vi "VISA init.vi"(8 "error in (no error)":errorcluster, 11 "UI Actor in":refnum<class "UI Actor.lvclass">) -> (0 "error out":errorcluster, 3 "UI Actor out":refnum<class "UI Actor.lvclass">)   [LabVIEW 2020, in "UI Actor.lvlib" / "UI Actor.lvclass"]
uses:
  UI Actor.lvclass
  UI Actor.lvclass/UI Actor.ctl
  Write VISA resource name.vi
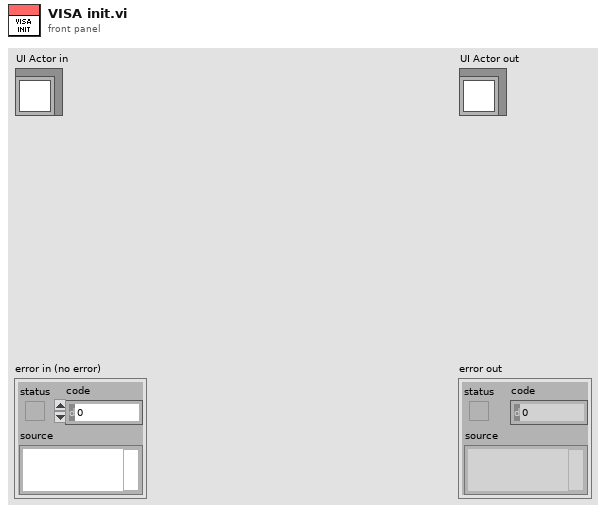
[diagram p1: front panel]
types:
  T1 = enum16{"Write", "Read", "Config", "Reset", "Close"}
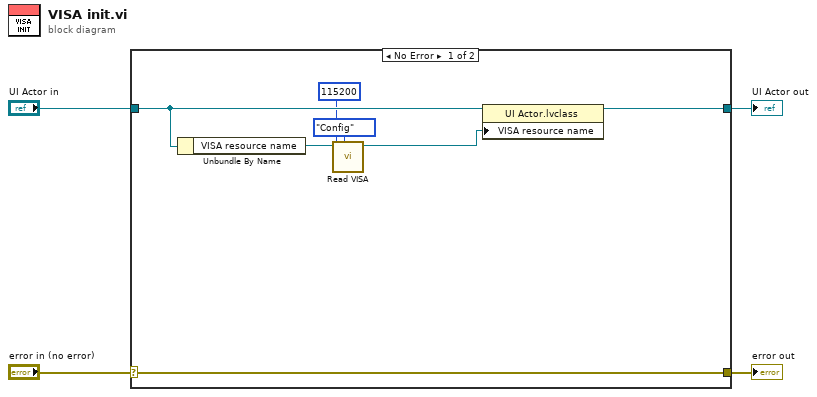
[diagram p0: block diagram]
diagram:
  n1 = case shown="No Error" "error in (no error)" {
    selector: "error in (no error)" -> [w11 w13]
    tunnel: [w11 w13] -> w3
    tunnel: [w6 w12] -> w1
    tunnel: "UI Actor in" -> [w10 w12]
    frame No Error {
      n2 = Unbundle By Name(w10) -> ("VISA resource name"=w9:refnum<visa-resource-name>)
      n3 = call "Read VISA.vi"("Opciones"=T1."Config", "baud rate (9600)"=u32 115200, "VISA com port"=w9) -> ("VISA com port 2"=w5:refnum<visa-resource-name>)  [unwired: 6 in, 2 out]
      n4 = property class="UI Actor.lvclass"(reference=w10, "VISA resource name"=w5) -> (reference out=w6:refnum<class "UI Actor.lvclass">)  [unwired: 1 in, 1 out]
    }
    frame Error {
    }
  }
  "error out" <- w3
  "UI Actor out" <- w1
